vi "Register UI Stop Event.vi"(8 "error in":errorcluster, 10 "Stop Button [ref]":refnum<vi>, 11 "Server Stop":refnum<user-event>) -> (0 "error out":errorcluster)   [LabVIEW 2020, in "MeasurementLink Measurement Server.lvlib"]
uses:
  <vilib>/MeasurementLink/MeasurementLink Measurement Server/MeasurementLink Measurement Server.lvlib
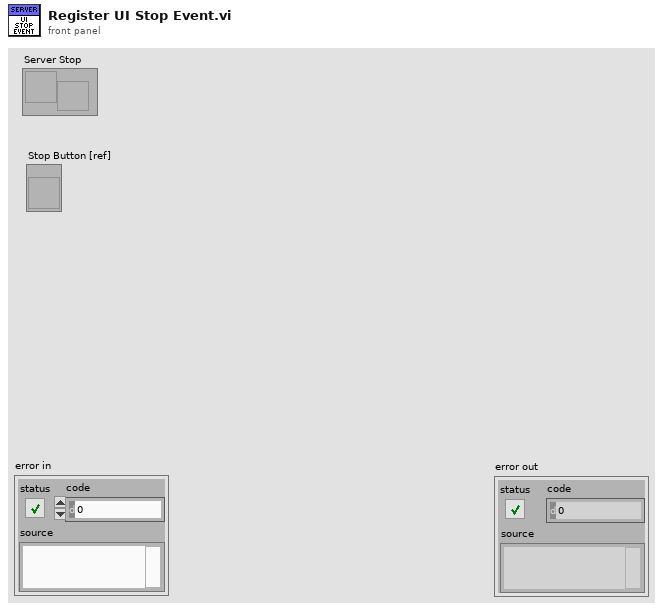
[diagram p1: front panel]
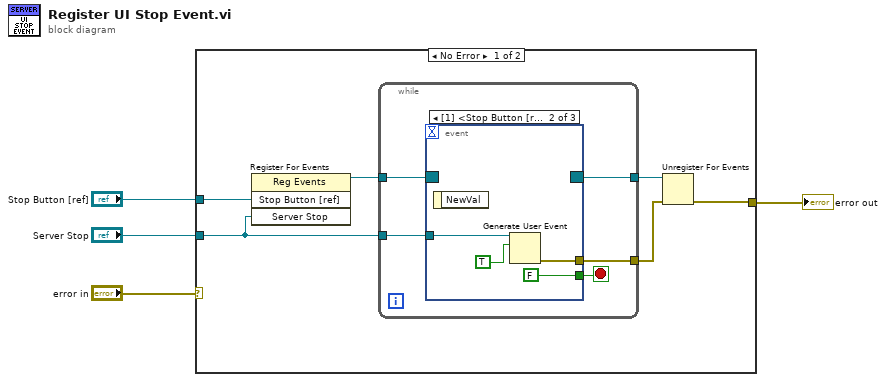
[diagram p0: block diagram]
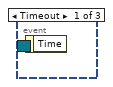
[diagram p2: hidden frame]
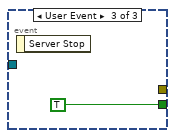
[diagram p3: hidden frame]
diagram:
  n1 = case shown="No Error" "error in" {
    selector: "error in" -> [_ w21]
    tunnel: [w5 w21] -> w4
    tunnel: "Stop Button [ref]" -> [w7 _]
    tunnel: "Server Stop" -> [w6 _]
    frame No Error {
      n2 = register-events(w7, w6) -> (reference out=w10:refnum<event-registration>)  [unwired: 2 in, 1 out]
      n3 = while {
        tunnel: w10 -> [w15]
        tunnel: [w13] -> w9
        tunnel: [w11] -> w8
        tunnel: w6 -> [w12]
        stop <- w14 stop-if-true
        n4 = event shown="[1] <Stop Button [ref]>: Value Change" {
          selector: w15 -> [_ _ _]
          dyn-events: [_ _ _] -> w13
          timeout: _ -> [_ _ _]
          tunnel: [_ FALSE TRUE] -> w14
          tunnel: w12 -> [_ w18 _]
          tunnel: [_ w16 _] -> w11
          event Timeout {
            n5 = event-data() -> ()  [unwired: 1 in, 1 out]
          }
          event Value Change {
            n6 = event-data() -> ()  [unwired: 1 in, 1 out]
            n7 = Generate User Event(user event=w18, event data cluster=TRUE ("event data")) -> (error out=w16:errorcluster)  [unwired: 2 in, 1 out]
          }
          event User Event {
            n8 = event-data() -> ()  [unwired: 1 in, 1 out]
          }
        }
      }
      n9 = Unregister For Events(event registration refnum=w9, error in=w8) -> (error out=w5:errorcluster)
    }
    frame Error {
    }
  }
  "error out" <- w4
